vi "stim config array refnum split (sub-vi).vi"(8 "error in (no error)":errorcluster, 11 "stim. config array refnum":refnum<vi>) -> (0 "error out":errorcluster, 2 "element refnum cluster":T1, 3 "stim. config array refnum out":refnum<vi>)   [LabVIEW 2021]
uses:
  type-defs/stimulation configuration array (type def).ctl
  type-defs/stimulator configuration line cluster (type def).ctl
  type-defs/port-odor with color cluster (type def).ctl
  type-defs/port-odor ring (type def).ctl
  type-defs/odor color (type def).ctl
panel:
  in  "stim. config array":T2 {"right odor"."port-odor ring" items=["off"]; "middle odor"."port-odor ring" items=["off"]; "left odor"."port-odor ring" items=["off"]}
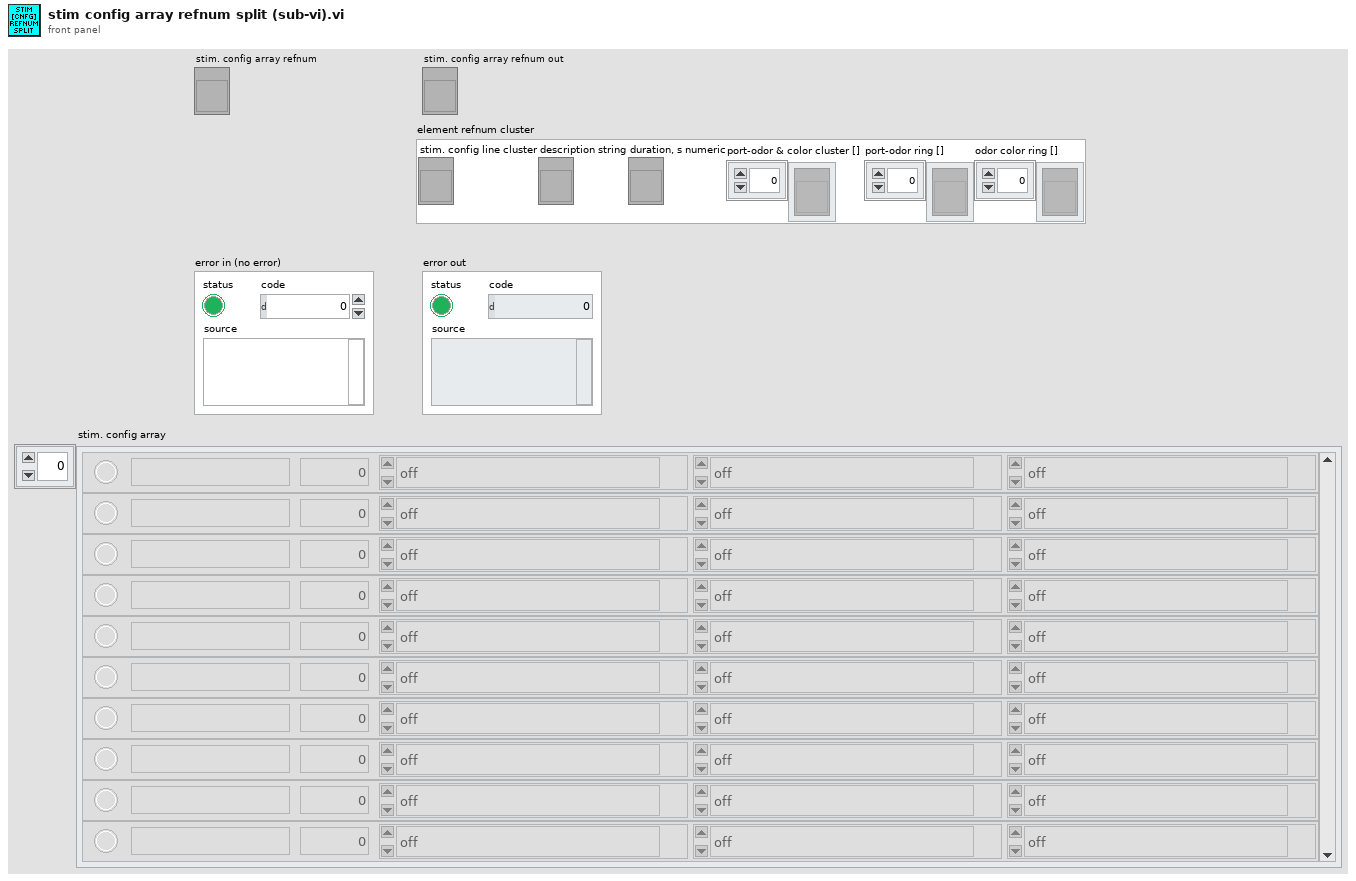
[diagram p1: front panel]
types:
  T1 = cluster{"stim. config line cluster":refnum<vi>, "description string":refnum<vi>, "duration, s numeric":refnum<vi>, "port-odor & color cluster []":refnum<vi>[], "port-odor ring []":refnum<vi>[], "odor color ring []":refnum<vi>[]}
  T2 = typedef "stimulation configuration array (type def).ctl" = T3[]
  T3 = typedef "stimulator configuration line cluster (type def).ctl" = cluster{"description":string, "duration, s":dbl, "left odor":T4, "middle odor":T4, "right odor":T4, "selected?":bool}
  T4 = typedef "port-odor with color cluster (type def).ctl" = cluster{"port-odor ring":T5, "odor color":T6}
  T5 = typedef "port-odor ring (type def).ctl" = u16
  T6 = typedef "odor color (type def).ctl" = u16
  T7 = cluster{"description string":refnum<vi>, "duration, s numeric":refnum<vi>, "port-odor & color cluster []":refnum<vi>[], "port-odor ring []":refnum<vi>[], "odor color ring []":refnum<vi>[]}
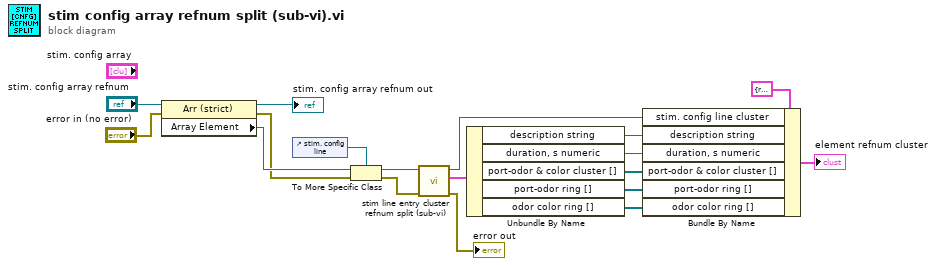
[diagram p0: block diagram]
diagram:
  n1 = property class="Arr (strict)"(reference="stim. config array refnum", error in="error in (no error)") -> (reference out=→"stim. config array refnum out":refnum<vi>, error out=w15:errorcluster, "Array Element"=w16:refnum<vi>)
  n2 = control-ref of="stim. config line"() -> (w14:refnum<vi>)
  n3 = To More Specific Class(target class=w14, reference=w16, error in=w15) -> (specific class reference=w12:refnum<vi>, error out=w11:errorcluster)
  n4 = call "stim line entry cluster refnum split (sub-vi).vi"("error in (no error)"=w11, "stim. config line cluster refnum"=w12) -> ("error out"=→"error out":errorcluster, "element refnum cluster"=w10:T7, "stim. config line cluster refnum out"=w4:refnum<vi>)  [unwired: 7 in]
  n5 = Unbundle By Name(w10) -> ("description string"=w9:refnum<vi>, "duration, s numeric"=w8:refnum<vi>, "port-odor & color cluster []"=w7:refnum<vi>[], "port-odor ring []"=w6:refnum<vi>[], "odor color ring []"=w5:refnum<vi>[])
  n6 = Bundle By Name(cluster=T1 {"stim. config line cluster"=refnum, "description string"=refnum, "duration, s numeric"=refnum, "port-odor & color cluster []"=[refnum, refnum, refnum], "port-odor ring []"=[refnum, refnum, refnum], "odor color ring []"=[refnum, refnum, refnum]} ("element refnum cluster"), "stim. config line cluster"=w4, "description string"=w9, "duration, s numeric"=w8, "port-odor & color cluster []"=w7, "port-odor ring []"=w6, "odor color ring []"=w5) -> (→"element refnum cluster":T1)
